vi "Generate Report.vi"(8 "error in (no error)":errorcluster, 11 "Data":variant) -> (0 "error out":errorcluster)   [LabVIEW 2014]
doc: "This subVI enqueues the named action in to the communications queue along with the input data."
uses:
  Private Controls/Module Action.ctl
  File IO.lvlib
  Private Controls/Module Data.ctl
panel:
  in  "Action":T1=enum."Generate Report"
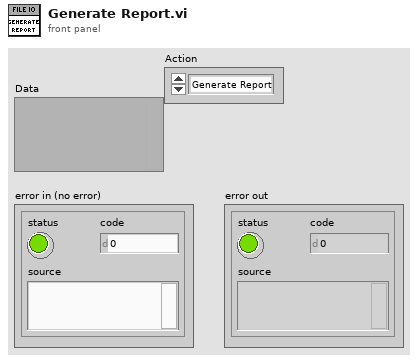
[diagram p1: front panel]
types:
  T1 = typedef "File IO.lvlib/Module Action.ctl" = enum8{"Init", "Error", "Exit", "CreateOpen Data File", "Write to Data File", "Generate Report", "Close Data File", "Open Admin Tools", "Load APU Setup File", "Save Calibration Data", "Crash Log", "Save APU Data", "Testing Type Select", "Set Testing State", "Set Recording State", "Check for Data", "Set Test Information", "Set Username", "Set Sample Rate", "Write System Log to File", "Increment Run Count", "Read Run Count"}
  T2 = typedef "File IO.lvlib/Module Data.ctl" = cluster{"Data":variant, "Action":T3}
  T3 = typedef "File IO.lvlib/Module Action.ctl" = enum8{"Init", "Error", "Exit", "CreateOpen Data File", "Open Admin Tools", "Save Calibration Data", "Crash Log", "Testing Type Select", "Set Testing State", "Set Recording State", "Set Test Information", "Set Sample Rate", "Set Username", "-----------Reporting-----------", "-------------TDMS -------------", "Check for Data", "Close Data File", "Add to System Log", "----------APU Setup File--------", "Save Stored APU Data", "Load APU Setup File", "Increment Run Count", "Write To Report", "Flush TDMS to File", "Create Report", "Set Report Filepath"}
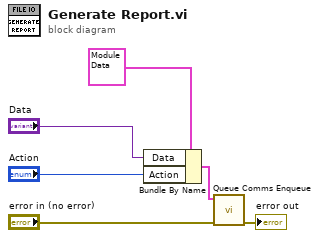
[diagram p0: block diagram]
diagram:
  n1 = Bundle By Name(cluster=T2 {"Data"=variant, "Action"=enum."Init"} ("element"), "Data"="Data", "Action"="Action") -> (w5:T2)
  n2 = call "Queue Comms Enqueue.vi"("error in (no error)"="error in (no error)", "element"=w5) -> ("error out"=→"error out":errorcluster)  [unwired: 9 in]
